vi "He3_Globals.vi"() -> ()   [LabVIEW 2013]
panel:
  out "Mini":dbl
  out "Main":dbl
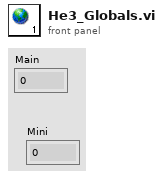
[diagram p1: front panel]
diagram:
